vi "LDO_Ultramat_23.vi"(8 "error in":errorcluster, 10 "VISA resource name":refnum<visa-resource-name>="OXYMAT", 11 "Message Queues":T1) -> (0 "error out":errorcluster)   [LabVIEW 2020]
uses:
  Message Queue/All Message Queues.ctl
  Message Queue/Message Cluster.ctl
  Message Queue/Enqueue Message (Single).vi
  Message Queue/Message Queue.lvlib
panel:
  out "Loop Count":i32
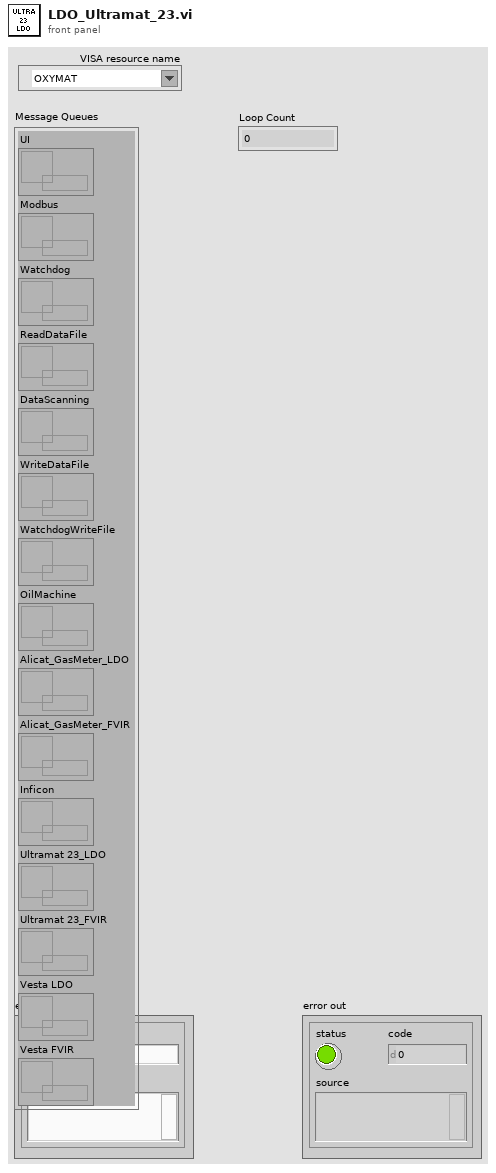
[diagram p1: front panel]
types:
  T1 = typedef "Message Queue.lvlib/All Message Queues.ctl" = cluster{"UI":refnum<queue>, "Modbus":refnum<queue>, "Watchdog":refnum<queue>, "ReadDataFile":refnum<queue>, "DataScanning":refnum<queue>, "WriteDataFile":refnum<queue>, "WatchdogWriteFile":refnum<queue>, "OilMachine":refnum<queue>, "Alicat_GasMeter_LDO":refnum<queue>, "Inficon":refnum<queue>, "Ultramat 23_LDO":refnum<queue>, "Alicat_GasMeter_FVIR":refnum<queue>, "Ultramat 23_FVIR":refnum<queue>, "Vesta LDO":refnum<queue>, "Vesta FVIR":refnum<queue>}
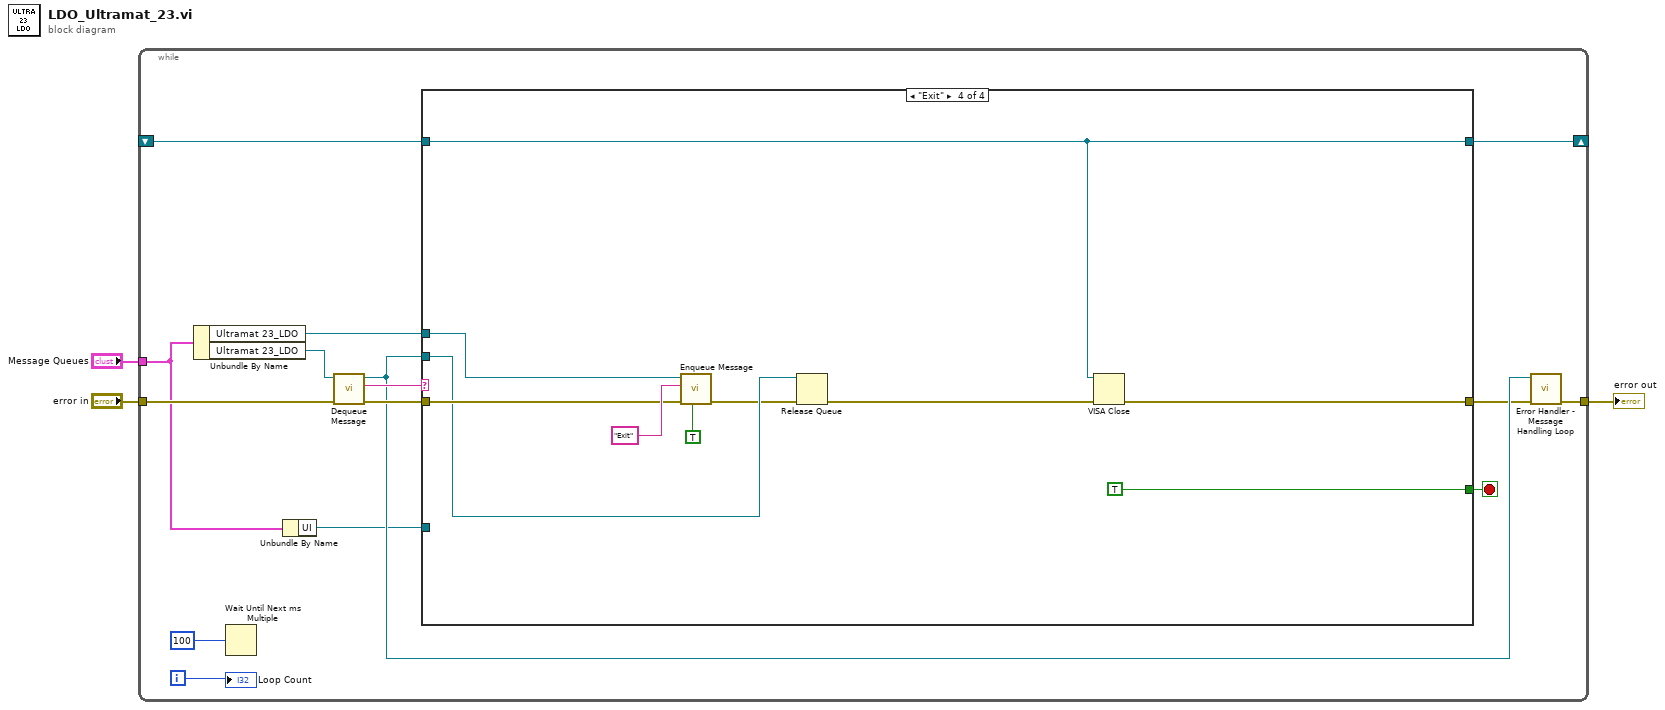
[diagram p0: block diagram]
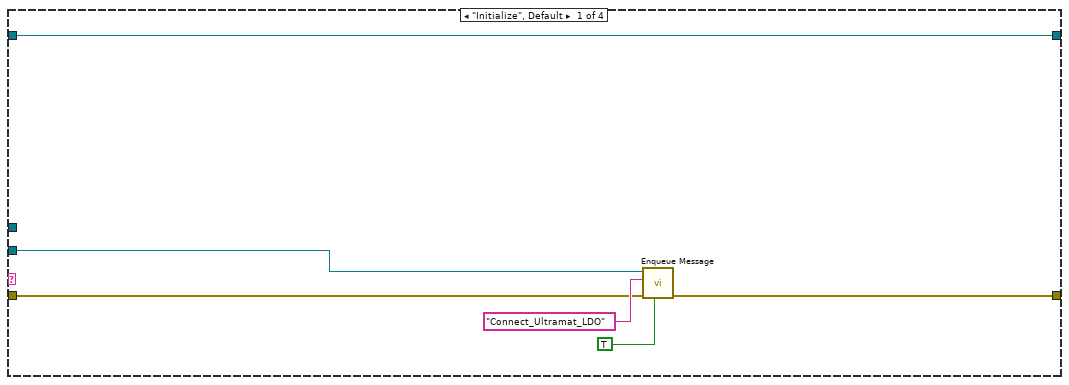
[diagram p2: hidden frame]
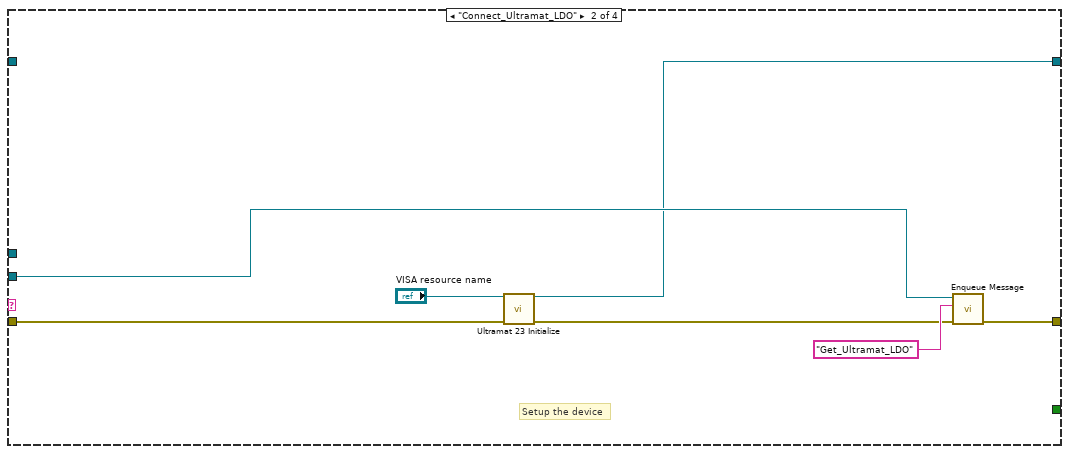
[diagram p3: hidden frame]
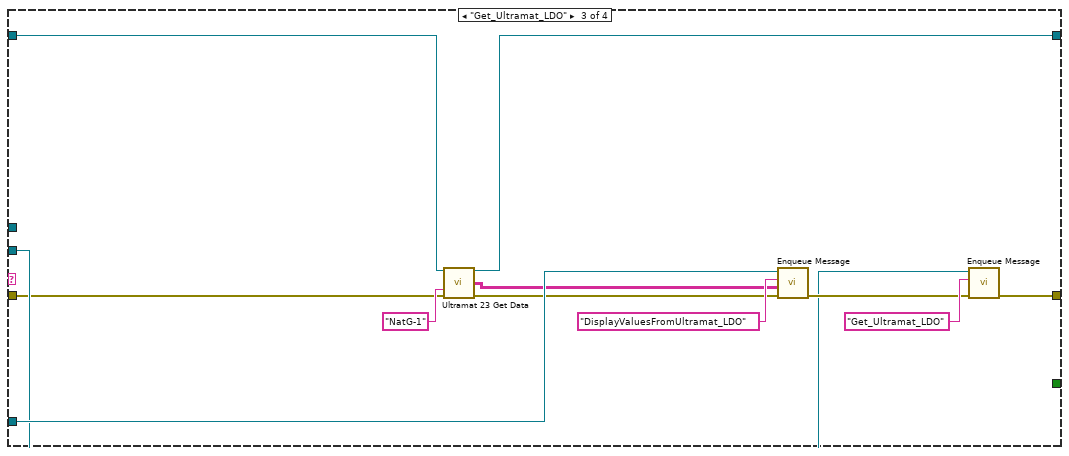
[diagram p4: hidden frame]
diagram:
  n1 = while {
    tunnel: "Message Queues" -> [w8]
    tunnel: "error in" -> [w17]
    tunnel: [w11] -> w1
    shift-right: [w6] -> _
    shift-left: _ -> [w5]
    i -> [w4]
    stop <- w14 stop-if-true
    n2 = Unbundle By Name(w8) -> ("Ultramat 23_LDO"=w13:refnum<queue>, "Ultramat 23_LDO"=w18:refnum<queue>)
    n3 = Wait Until Next ms Multiple(millisecond multiple=u32 100) -> ()  [unwired: 1 out]
    n4 = Unbundle By Name(w8) -> ("UI"=w7:refnum<queue>)
    n5 = call "Dequeue Message.vi"("error in (no error)"=w17, "Message Queue"=w18) -> ("error out"=w15:errorcluster, "Message"=w16:string, "dup Message Queue"=w12:refnum<queue>)  [unwired: 6 in, 1 out]
    n6 = case shown="\"Exit\"" w16 {
      tunnel: w15 -> [w23 w28 w32 w49]
      tunnel: [w22 w30 w39 w45] -> w10
      tunnel: [_ _ _ TRUE] -> w14
      tunnel: w13 -> [_ _ _ w50]
      tunnel: w12 -> [w21 w29 w38 w48]
      tunnel: w7 -> [_ _ w42 _]
      tunnel: [w20 w25 w35 w44] -> w6
      tunnel: w5 -> [w20 _ w36 w44]
      frame "Initialize", Default {
        n7 = call-poly "Enqueue Message.vi"("Priority Message? (F)"=TRUE, "error in (no error)"=w23, "Message"="Connect_Ultramat_LDO", "Message Queue"=w21) -> ("error out"=w22:errorcluster)  [unwired: 6 in, 1 out]
      }
      frame "Connect_Ultramat_LDO" {
        # "Setup the device"
        n8 = call "Ultramat 23 Initialize.vi"("VISA resource name"="VISA resource name", "error in (no error)"=w28) -> ("VISA Session Out"=w25:refnum<visa-resource-name>, "error out"=w27:errorcluster)  [unwired: 8 in, 4 out]
        n9 = call-poly "Enqueue Message.vi"("error in (no error)"=w27, "Message"="Get_Ultramat_LDO", "Message Queue"=w29) -> ("error out"=w30:errorcluster)  [unwired: 7 in, 1 out]
      }
      frame "Get_Ultramat_LDO" {
        n10 = call "Ultramat 23 Get Data.vi"("VISA resource name"=w36, "Gas selected"="NatG-1", "error in (no error)"=w32) -> ("VISA Session Out"=w35:refnum<visa-resource-name>, "Data Array"=w34:string[][], "error out"=w37:errorcluster)  [unwired: 8 in, 2 out]
        n11 = call-poly "Enqueue Message.vi"("error in (no error)"=w37, "Message Data"=w34, "Message"="DisplayValuesFromUltramat_LDO", "Message Queue"=w42) -> ("error out"=w40:errorcluster)  [unwired: 6 in, 1 out]
        n12 = call-poly "Enqueue Message.vi"("error in (no error)"=w40, "Message"="Get_Ultramat_LDO", "Message Queue"=w38) -> ("error out"=w39:errorcluster)  [unwired: 7 in, 1 out]
      }
      frame "Exit" {
        n13 = call-poly "Enqueue Message.vi"("Priority Message? (F)"=TRUE, "error in (no error)"=w49, "Message"="Exit", "Message Queue"=w50) -> ("error out"=w47:errorcluster)  [unwired: 6 in, 1 out]
        n14 = Release Queue(queue=w48, error in (no error)=w47) -> (error out=w46:errorcluster)  [unwired: 1 in, 2 out]
        n15 = VISA Close(VISA resource name=w44, error in (no error)=w46) -> (error out=w45:errorcluster)
      }
    }
    n16 = call "Error Handler - Message Handling Loop.vi"("error in (no error)"=w10, "Message Queue"=w12) -> ("dup error in"=w11:errorcluster)  [unwired: 8 in, 1 out]
    "Loop Count" <- w4
  }
  "error out" <- w1
